vi "Load Scan from File Path.vi"(6 "TreeControl in":refnum<vi>, 7 "Data Cluster In":T1={"Project"=refnum, "Current Selection"={"Library"=refnum, "VI"=refnum}, "Module ID"=-1, "Tree Selection"=""}, 8 "error in":errorcluster, 11 "Project Path":path=path "C:/Users/Enrique Noé Arias/Desktop/Untitled Project 1/PantherScan.xml") -> (0 "error out":errorcluster, 2 "Continue?":bool, 5 "Data Cluster Out":T1={"Project"=refnum, "Current Selection"={"Library"=refnum, "VI"=refnum}, "Module ID"=-1, "Tree Selection"=""})   [LabVIEW 2020, in "Panther Dashboard.lvlib"]
doc: "Gets the Singleton and Cloneable references and creates a list of each type of DQMH Modules"
uses:
  Panther Dashboard.lvlib
  Module Data--cluster.ctl
  Class/Project/Project.lvclass
  Class/Library/Library.lvclass
  Class/VI/VI.lvclass
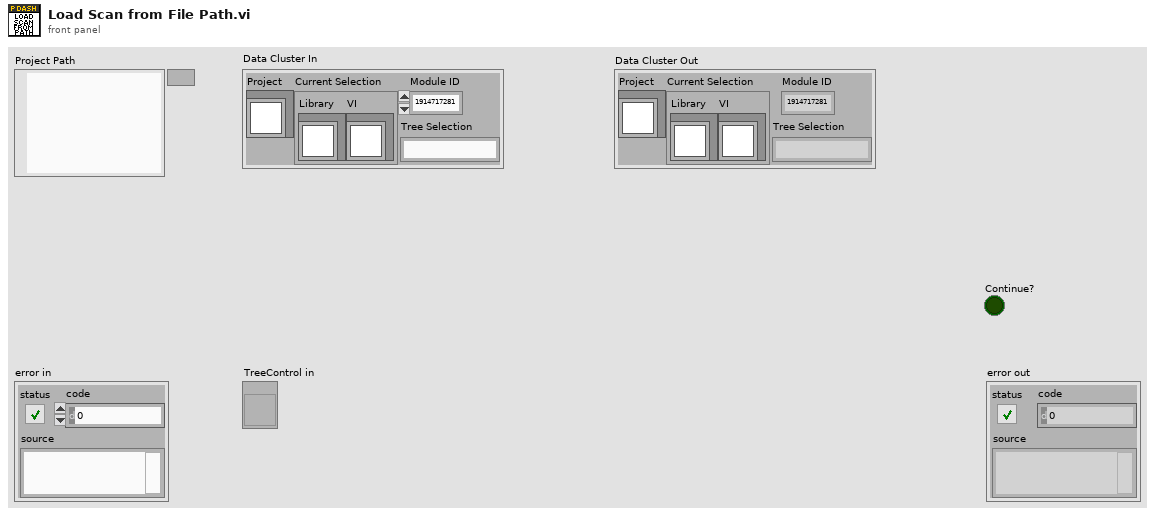
[diagram p1: front panel]
types:
  T1 = typedef "Panther Dashboard.lvlib/Module Data--cluster.ctl" = cluster{"Project":refnum<class "Project.lvclass">, "Current Selection":cluster{"Library":refnum<class "Library.lvclass">, "VI":refnum<class "VI.lvclass">}, "Module ID":i32, "Tree Selection":string}
  T2 = typedef "Tree Map.lvlib/Tree Map Data.ctl" = map{string, cluster{"Child Paths Set":set{string}, "Name":string, "Data":string, "Attributes":map{string, string}}}
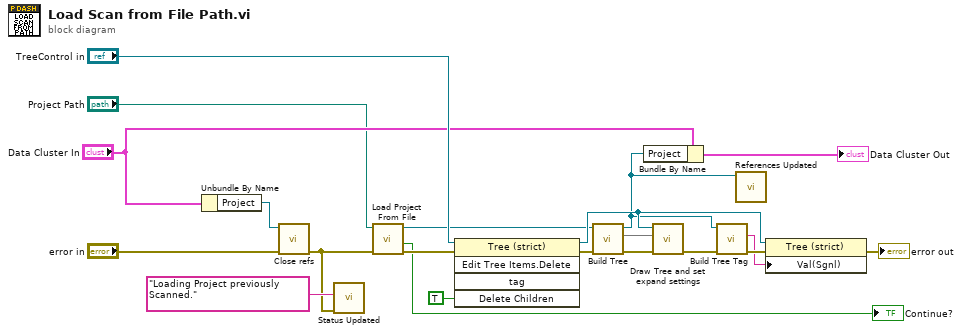
[diagram p0: block diagram]
diagram:
  n1 = Unbundle By Name("Data Cluster In") -> ("Project"=w13:refnum<class "Project.lvclass">)
  n2 = call "Close refs.vi"("error in"="error in", "Project"=w13) -> ("error out"=w1:errorcluster)  [unwired: 9 in]
  n3 = call "Status Updated.vi"("error in (no error)"=w1, "Status"="Loading Project previously Scanned.") -> ()  [unwired: 9 in, 1 out]
  n4 = call "Load Project From File.vi"("error in"=w1, "Project Path"="Project Path") -> ("error out"=w20:errorcluster, "Continue?"=→"Continue?":bool, "Project out"=w5:refnum<class "Project.lvclass">)  [unwired: 7 in]
  n5 = invoke class="Tree (strict)" method="Edit Tree Items.Delete"(reference="TreeControl in", error in=w20, "Delete Children"=TRUE ("Delete Children?")) -> (reference out=w6:refnum<vi>, error out=w19:errorcluster)  [unwired: 2 in, 3 out]
  n6 = call "Build Tree.vi"("error in"=w19, "Project in"=w5) -> ("error out"=w18:errorcluster, "Tree Map Out"=w7:T2, "Project Out"=w3:refnum<class "Project.lvclass">)  [unwired: 7 in]
  n7 = Bundle By Name(cluster="Data Cluster In", "Project"=w3) -> (→"Data Cluster Out":T1)
  n8 = call "Draw Tree and set expand settings.vi"("error in"=w18, "Tree Map In"=w7, "TreeControl in"=w6) -> ("error out"=w17:errorcluster)  [unwired: 8 in]
  n9 = call "Build Tree Tag.vi"("error in"=w17, "Project"=w3) -> ("error out"=w16:errorcluster, "Tree Tag"=w4:string)  [unwired: 8 in]
  n10 = call "References Updated.vi"("Project"=w3) -> ()  [unwired: 10 in, 1 out]
  n11 = property class="Tree (strict)"(reference=w6, error in=w16, "Val(Sgnl)"=w4) -> (error out=→"error out":errorcluster)  [unwired: 1 out]
